vi "Stop Core.vi"(10 "final error code":i32, 11 "VIStore in":refnum<class "StoreUI.lvclass">) -> (3 "VIStore out":refnum<class "StoreUI.lvclass">)   [LabVIEW 2015, in "StoreUI.lvlib" / "StoreUI.lvclass"]
doc: "(<B>Filename</B>: Actor Framework.lvlib:Actor.lvclass:Stop Core.vi)\n\nDefines what the actor does before it stops. Use the <B>final error code</B> input to determine whether the actor shut down in response to an error.\n\nBy default, this method does nothing. A descendant class may override it to define behavior, such as shutting down any processes the actor initiated in its override of the Actor Core method."
uses:
  StoreUI.lvclass
  StoreUI.lvclass/StoreUI.ctl
  <vilib>/ActorFramework/Message Enqueuer/Message Enqueuer.lvclass/Message Enqueuer.ctl
  <vilib>/ActorFramework/Message Enqueuer/Enqueue.vi
  <vilib>/ActorFramework/Message Priority Queue/Priority Enqueue.vi
  <vilib>/ActorFramework/Stop Msg/Stop Msg.lvclass
  <vilib>/ActorFramework/Actor/Actor.lvclass
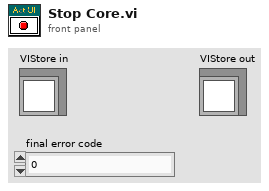
[diagram p1: front panel]
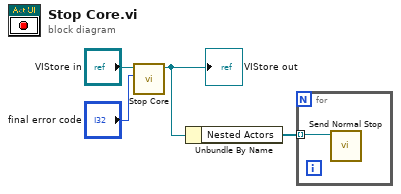
[diagram p0: block diagram]
diagram:
  n1 = call-parent "Stop Core.vi"("final error code"="final error code", "Actor in"="VIStore in") -> ("Actor out"=w2:refnum<class "StoreUI.lvclass">)  [unwired: 9 in]
  "VIStore out" <- w2
  n2 = Unbundle By Name(w2) -> ("Nested Actors"=w1:refnum<class "Message Enqueuer.lvclass">[])
  n3 = for {
    tunnel: w1 -> [w5] mode=indexing
    n4 = call <vilib>:"Send Normal Stop.vi"("Message Enqueuer"=w5) -> ()  [unwired: 10 in, 1 out]
  }
